vi "Axis modifications.vi"(1 "Driver JoyStick Info":cluster{"Slow Drive?":bool, "Axisses":dbl[]}) -> (0 "Driver JoyStick Info Out":cluster{"Slow Drive?":bool, "Axisses":dbl[]})   [LabVIEW 2012]
uses:
  Drive Global Data.vi
panel:
  # "Out"
  # "In"
  # "X"
  # "Y"
  # "X"
  # "Y"
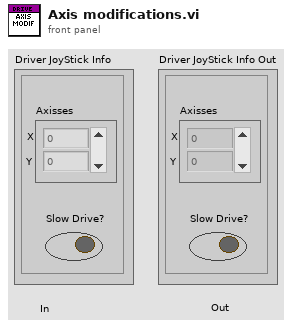
[diagram p1: front panel]
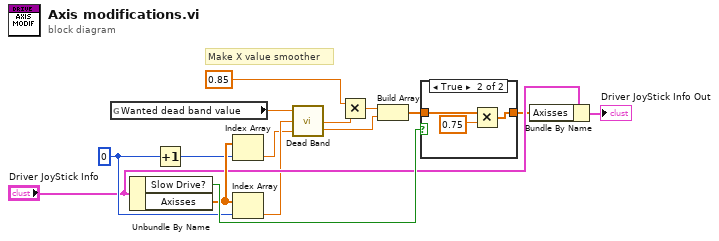
[diagram p0: block diagram]
diagram:
  w12 = 0 ("index")
  # "Make X value smoother"
  n1 = global read "Drive Global Data.vi" "Wanted dead band value"() -> (w5:dbl)
  n2 = Unbundle By Name("Driver JoyStick Info") -> ("Slow Drive?"=w15:bool, "Axisses"=w14:dbl[])
  n3 = Increment(x=w12) -> (x+1=w13:i32)
  n4 = Index Array(array=w14, index=w13) -> (element=w7:dbl)
  n5 = Index Array(array=w14, index=w12) -> (element=w8:dbl)
  n6 = call "Dead Band.vi"("Axis 2 In"=w7, "Axis 1 In"=w8, "Dead Band"=w5) -> ("Axis 2 Out"=w3:dbl, "Axis 1 Out"=w6:dbl)
  n7 = Multiply(x=0.85, y=w6) -> (x*y=w4:dbl)
  n8 = Build Array(w4, w3) -> (w2:dbl[])
  n9 = case shown="True" w15 {
    tunnel: [w16 w18] -> w1
    tunnel: w2 -> [w16 w17]
    frame False {
    }
    frame True {
      n10 = Multiply(x=w17, y=0.75) -> (x*y=w18:dbl[])
    }
  }
  n11 = Bundle By Name(cluster="Driver JoyStick Info", "Axisses"=w1) -> (→"Driver JoyStick Info Out":cluster{"Slow Drive?":bool, "Axisses":dbl[]})
